vi "Init Kinect.vi"() -> ()   [LabVIEW 2011]
uses:
  Microsoft.Kinect
  Kinect Global Status.vi
panel:
  in  "Depth Format":i32(ring)=1 items=["Undefined", "Resolution640x480Fps30", "Resolution320x240Fps30", "Resolution80x60Fps30"]
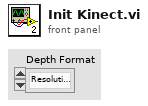
[diagram p1: front panel]
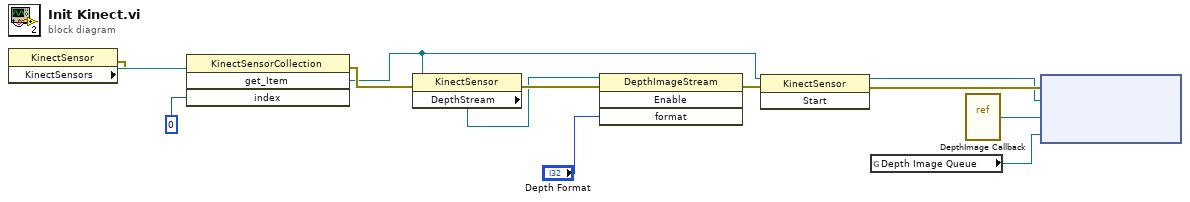
[diagram p0: block diagram]
diagram:
  n1 = property class="KinectSensor"() -> (error out=w11:errorcluster, "KinectSensors"=w13:refnum<k24>)  [unwired: 2 in, 1 out]
  n2 = invoke class="KinectSensorCollection" method="get_Item"(reference=w13, error in=w11, "index"=0) -> (error out=w10:errorcluster, "get_Item"=w6:refnum<k24>)  [unwired: 1 in, 2 out]
  n3 = property class="KinectSensor"(reference=w6, error in=w10) -> (error out=w9:errorcluster, "DepthStream"=w5:refnum<k24>)  [unwired: 1 out]
  n4 = invoke class="DepthImageStream" method="Enable"(reference=w5, error in=w9, "format"="Depth Format") -> (error out=w8:errorcluster)  [unwired: 1 in, 3 out]
  n5 = invoke class="KinectSensor" method="Start"(reference=w6, error in=w8) -> (reference out=w2:refnum<k24>, error out=w3:errorcluster)  [unwired: 1 in, 1 out]
  n6 = global read "Kinect Global Status.vi" "Depth Image Queue"() -> (w4:refnum<queue>)
  n7 = vi-ref "DepthImage Callback.vi"() -> ("vi reference"=w1:refnum<vi>)
  n8 = node(w3, w2, w1, w4) -> ()  [unwired: 1 in, 2 out]
